vi "Subpanel Visibility.vi"(5 "Maximized?":bool, 7 "Visible":bool, 8 "error in (no error)":errorcluster, 10 "Panel":T1 {"Plot Bounds (%)"."Bottom (%)" format="%.2f"; "Plot Bounds (%)"."Top (%)" format="%.2f"; "Plot Bounds (%)"."Right (%)" format="%.2f"; "Plot Bounds (%)"."Left (%)" format="%.2f"}, 11 "Manager in":refnum<class "Manager.lvclass">) -> (0 "error out":errorcluster, 3 "Manager out":refnum<class "Manager.lvclass">)   [LabVIEW 2021, in "MultiRocketPlotPanel.lvclass"]
uses:
  MultiRocketPlotPanel.lvclass
  <vilib>/IlluminatedG/IG OOPanel/OOPanel/Manager/Manager.lvclass
  SubVIs/Panel Map Data.ctl
  <userlib>/bjustice/RocketPlot/Classes/RocketPlotPanel/RocketPlotPanel.lvclass
  SubVIs/Window Position.ctl
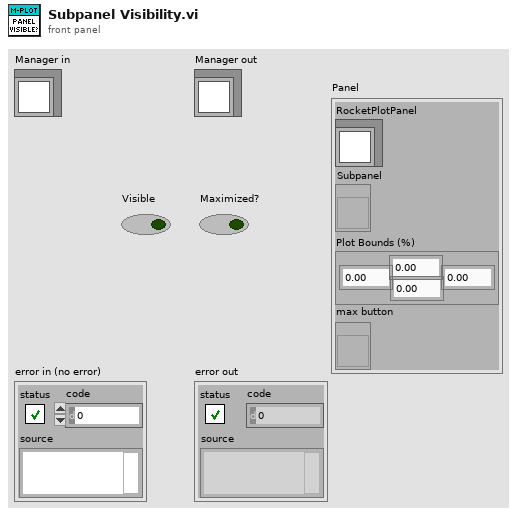
[diagram p1: front panel]
types:
  T1 = typedef "MultiRocketPlotPanel.lvclass/Panel Map Data.ctl" = cluster{"RocketPlotPanel":refnum<class "RocketPlotPanel.lvclass">, "Subpanel":refnum<vi>, "Plot Bounds (%)":T2, "max button":refnum<vi>}
  T2 = typedef "MultiRocketPlotPanel.lvclass/Window Position.ctl" = cluster{"Left (%)":dbl, "Top (%)":dbl, "Right (%)":dbl, "Bottom (%)":dbl}
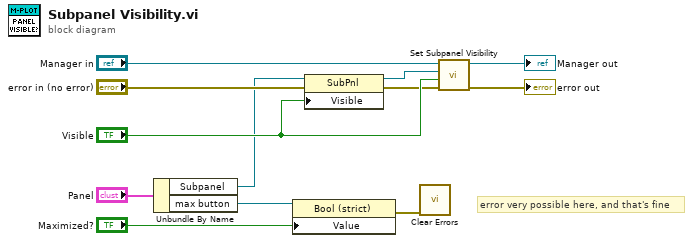
[diagram p0: block diagram]
diagram:
  # "error very possible here, and that's fine"
  n1 = Unbundle By Name("Panel") -> ("Subpanel"=w4:refnum<vi>, "max button"=w3:refnum<vi>)
  n2 = property class="Bool (strict)"(reference=w3, "Value"="Maximized?") -> (error out=w2:errorcluster)  [unwired: 1 in, 1 out]
  n3 = property class="SubPnl"(reference=w4, error in="error in (no error)", "Visible"="Visible") -> (reference out=w9:refnum<vi>, error out=w6:errorcluster)
  n4 = call <vilib>:"Clear Errors.vi"("error in (no error)"=w2) -> ()  [unwired: 5 in, 2 out]
  n5 = call <vilib>:"Set Subpanel Visibility.vi"("error in (no error)"=w6, "Visible"="Visible", "SubPanel"=w9, "Manager in"="Manager in") -> ("error out"=→"error out":errorcluster, "Manager out"=→"Manager out":refnum<class "Manager.lvclass">)  [unwired: 6 in]
